vi "北斗参数配置.vi"() -> ()   [LabVIEW 2016, in "环境动力监测库.lvlib" / "NMEA.lvlib"]
uses:
  NMEA.lvlib
  <vilib>/Utility/config.llb/NI_LVConfig.lvlib
panel:
  in  "收方地址设定值":string
  in  "移位报警设定值":dbl=1000.0
  # "北斗参数配置"
  # "米"
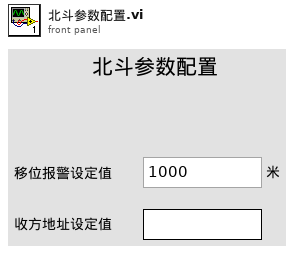
[diagram p1: front panel]
types:
  T1 = typedef "NI_LVConfig.lvlib/Config Data RefNum.ctl" = refnum<k1>
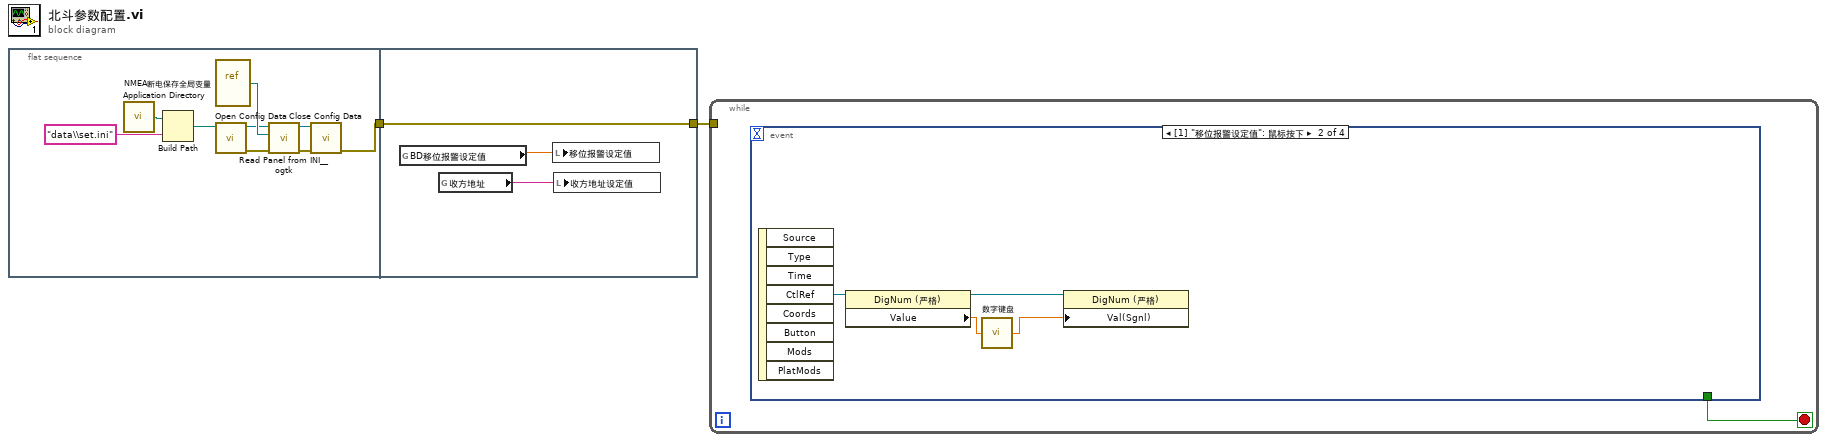
[diagram p0: block diagram]
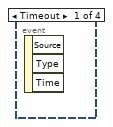
[diagram p2: hidden frame]
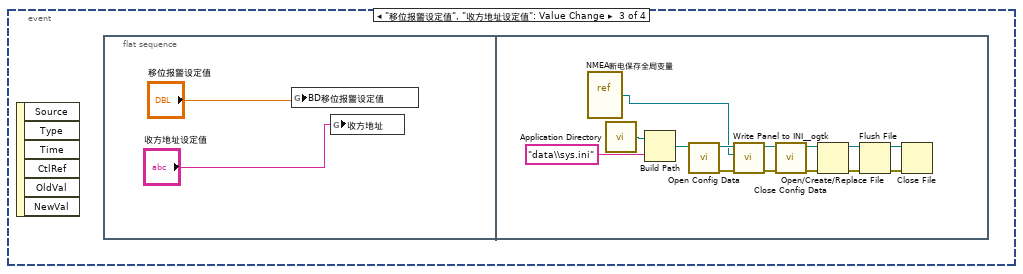
[diagram p3: hidden frame]
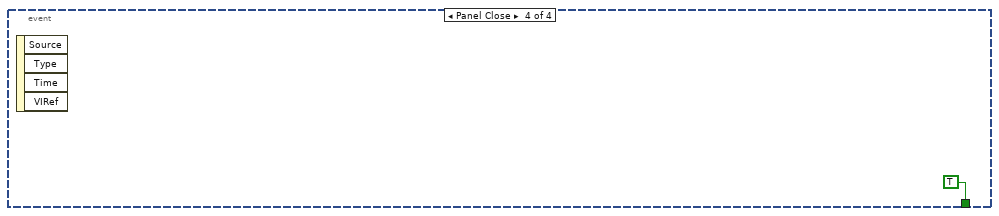
[diagram p4: hidden frame]
diagram:
  n1 = flat-sequence {
    tunnel: [w3] -> w2
    tunnel: [w14] -> w1
    tunnel: w2 -> [w14]
    frame #0 {
      n2 = call <vilib>:"Application Directory.vi"() -> ("Application Directory"=w9:path)
      n3 = Build Path(base path=w9, name or relative path="data\\set.ini" ("名称或相对路径")) -> (appended path=w10:path)
      n4 = vi-ref "NMEA断电保存全局变量.vi"() -> (w11:refnum<vi>)
      n5 = call <vilib>:"Open Config Data.vi"("configuration file path"=w10) -> ("error out"=w6:errorcluster, "refnum"=w7:T1)  [unwired: 8 in, 1 out]
      n6 = call <userlib>:"Read Panel from INI__ogtk.vi"("error in (no error)"=w6, "VI ref"=w11, "refnum"=w7) -> ("error out"=w4:errorcluster, "refnum out"=w5:T1)  [unwired: 7 in]
      n7 = call <vilib>:"Close Config Data.vi"("error in (no error)"=w4, "refnum"=w5) -> ("error out"=w3:errorcluster)  [unwired: 8 in, 1 out]
    }
    frame #1 {
      n8 = global read "NMEA断电保存全局变量.vi" "BD移位报警设定值"() -> (w12:dbl)
      n9 = global read "NMEA断电保存全局变量.vi" "收方地址"() -> (w13:string)
      n10 = local write "移位报警设定值"(w12) -> ()
      n11 = local write "收方地址设定值"(w13) -> ()
    }
  }
  n12 = while {
    tunnel: w1 -> [_]
    stop <- w15 stop-if-true
    n13 = event shown="[1] \"移位报警设定值\": 鼠标按下" {
      selector: _ -> [_ _ _ _]
      dyn-events: _ -> [_ _ _ _]
      timeout: _ -> [_ _ _ _]
      tunnel: [_ _ _ TRUE] -> w15
      event Timeout {
        n14 = event-data() -> ()  [unwired: 1 in, 3 out]
      }
      event "移位报警设定值": Mouse Down {
        n15 = event-data() -> ("CtlRef"=w16:refnum<vi>)  [unwired: 1 in, 7 out]
        n16 = property class="DigNum (严格)"(reference=w16) -> (reference out=w18:refnum<vi>, "Value"=w19:dbl)  [unwired: 1 in, 1 out]
        n17 = call "数字键盘.vi"("OldNumber"=w19) -> ("NewNumber"=w17:sgl)
        n18 = property class="DigNum (严格)"(reference=w18, "Val(Sgnl)"=w17) -> ()  [unwired: 1 in, 2 out]
      }
      event "移位报警设定值", "收方地址设定值": Value Change {
        n19 = event-data() -> ()  [unwired: 1 in, 6 out]
        n20 = flat-sequence {
          frame #0 {
            n21 = global write "NMEA断电保存全局变量.vi" "BD移位报警设定值"("移位报警设定值") -> ()
            n22 = global write "NMEA断电保存全局变量.vi" "收方地址"("收方地址设定值") -> ()
          }
          frame #1 {
            n23 = vi-ref "NMEA断电保存全局变量.vi"() -> (w22:refnum<vi>)
            n24 = call <vilib>:"Application Directory.vi"() -> ("Application Directory"=w35:path)
            n25 = Build Path(base path=w35, name or relative path="data\\sys.ini" ("名称或相对路径")) -> (appended path=w33:path)
            n26 = call <vilib>:"Open Config Data.vi"("configuration file path"=w33) -> ("error out"=w30:errorcluster, "refnum"=w32:T1)  [unwired: 8 in, 1 out]
            n27 = call <userlib>:"Write Panel to INI__ogtk.vi"("error in (no error)"=w30, "VI ref"=w22, "refnum"=w32) -> ("error out"=w29:errorcluster, "refnum out"=w31:T1)  [unwired: 7 in]
            n28 = call <vilib>:"Close Config Data.vi"("error in (no error)"=w29, "refnum"=w31) -> ("error out"=w24:errorcluster, "file path"=w23:path)  [unwired: 8 in]
            n29 = Open/Create/Replace File(file path (use dialog)=w23, error in=w24) -> (refnum out=w27:refnum<file>, error out=w28:errorcluster)  [unwired: 4 in, 1 out]
            n30 = Flush File(refnum=w27, error in=w28) -> (refnum out=w26:refnum<file>, error out=w25:errorcluster)
            n31 = Close File(refnum=w26, error in=w25) -> ()  [unwired: 2 out]
          }
        }
      }
      event Panel Close {
        n32 = event-data() -> ()  [unwired: 1 in, 4 out]
      }
    }
  }
